vi "define.vi"(8 "error in (no error)":errorcluster, 11 "ColorOverlay in":refnum<class "ColorOverlay.lvclass">) -> (0 "error out":errorcluster, 2 "color cluster out":T2(array[cluster]), 3 "ColorOverlay out":refnum<class "ColorOverlay.lvclass">)   [LabVIEW 2010, in "ColorOverlay.lvclass"]
uses:
  ColorOverlay.lvclass
  <vilib>/Utility/miscctls.llb/LVPointTypeDef.ctl
  ColorOverlay.lvclass/ColorOverlay.ctl
  settings_cluster.ctl
  cursor_cluster.ctl
  enum_color_channel.ctl
panel:
  in  "presets":string(combo)
  in  "range":cluster{dbl, dbl}(slide)={255.0, 255.0} scale=1e-05..0.999999
  out "random image out":T1(plugin-control)
  in  "button: done":bool
  in  "color?":bool=TRUE
  in  "start color":cluster{dbl, dbl, dbl, dbl}(slide)={0.0, 0.0, 255.0, 0.0} scale=1e-10..255.0
  in  "end color":cluster{dbl, dbl, dbl, dbl}(slide)={255.0, 0.0, 0.0, 255.0} scale=1e-10..255.0
  in  "# cold pixels":i32 min=0 max=255
  in  "# hot pixels":i32 min=0 max=255
  in  "color lower limit":u32(colorbox)=16860
  in  "color upper limit":u32(colorbox)=16711680
  out "color bar":u32[](array[colorbox])
  out "graph editor":cluster{"ramp array out":u32[]}[](graph)=[{"ramp array out"=[0, 0, 0, 0, 0, 0, 0, 0, 0, 0, 0, 0, 0, 1, 1, 1, 1, 1, 1, 1, 1, 1, 1, 1, 1, 1, 1, 1, 1, 1, 1, 1, 1, 1, 1, 1, 1, 1, 1, 2, 2, 2, 2, 2, 2, 2, 2, 2, 2, 2, 2, 2, 2, 2, 2, 2, 2, 2, 2, 2, 2, 2, 2, 2, 3, 3, 3, 3, 3, 3, 3, 3, 3, 3, 3, 3, 3, 3, 3, 3, 3, 3, 3, 3, 3, 3, 3, 3, 3, 4, 4, 4, 4, 4, 4, 4, 4, 4, 4, 4, 4, 4, 4, 4, 4, 4, 4, 4, 4, 4, 4, 4, 4, 4, 4, 5, 5, 5, 5, 5, 5, 5, 5, 5, 5, 5, 5, 5, 7, 9, 11, 13, 15, 17, 19, 21, 22, 24, 26, 28, 30, 32, 34, 36, 38, 40, 42, 44, 46, 48, 50, 52, 53, 55, 57, 59, 61, 63, 65, 67, 69, 71, 73, 75, 77, 79, 81, 83, 84, 86, 88, 90, 92, 94, 96, 98, 100, 102, 104, 106, 108, 110, 112, 114, 115, 117, 119, 121, 123, 125, 127, 129, 131, 133, 135, 137, 139, 141, 143, 145, 146, 148, 150, 152, 154, 156, 158, 160, 162, 164, 166, 168, 170, 172, 174, 176, 177, 179, 181, 183, 185, 187, 189, 191, 193, 195, 197, 199, 201, 203, 205, 207, 208, 210, 212, 214, 216, 218, 220, 222, 224, 226, 228, 230, 232, 234, 236, 238, 239, 241, 243, 245, 247, 249, 251, 253]}, {"ramp array out"=[0, 2, 4, 6, 8, 10, 12, 14, 16, 18, 20, 22, 24, 26, 28, 30, 32, 34, 36, 38, 40, 42, 44, 46, 48, 50, 52, 54, 56, 58, 60, 62, 64, 66, 68, 70, 72, 74, 76, 78, 80, 82, 84, 86, 88, 90, 92, 94, 96, 98, 100, 102, 104, 106, 108, 110, 112, 114, 116, 118, 120, 122, 124, 126, 129, 131, 133, 135, 137, 139, 141, 143, 145, 147, 149, 151, 153, 155, 157, 159, 161, 163, 165, 167, 169, 171, 173, 175, 177, 179, 181, 183, 185, 187, 189, 191, 193, 195, 197, 199, 201, 203, 205, 207, 209, 211, 213, 215, 217, 219, 221, 223, 225, 227, 229, 231, 233, 235, 237, 239, 241, 243, 245, 247, 249, 251, 253, 255, 253, 251, 249, 247, 245, 243, 241, 239, 237, 235, 233, 231, 229, 227, 225, 223, 221, 219, 217, 215, 213, 212, 210, 208, 206, 204, 202, 200, 198, 196, 194, 192, 190, 188, 186, 184, 182, 180, 178, 176, 174, 172, 170, 168, 166, 164, 162, 160, 158, 156, 154, 152, 150, 148, 146, 144, 142, 140, 138, 136, 134, 132, 130, 128, 127, 125, 123, 121, 119, 117, 115, 113, 111, 109, 107, 105, 103, 101, 99, 97, 95, 93, 91, 89, 87, 85, 83, 81, 79, 77, 75, 73, 71, 69, 67, 65, 63, 61, 59, 57, 55, 53, 51, 49, 47, 45, 43, 42, 40, 38, 36, 34, 32, 30, 28, 26, 24, 22, 20, 18, 16, 14, 12, 10, 8, 6, 4, 2]}, {"ramp array out"=[255, 253, 251, 249, 247, 245, 243, 241, 239, 237, 235, 233, 231, 229, 227, 225, 224, 222, 220, 218, 216, 214, 212, 210, 208, 206, 204, 202, 200, 198, 196, 194, 192, 190, 188, 186, 184, 182, 180, 178, 176, 174, 172, 170, 168, 166, 164, 162, 161, 159, 157, 155, 153, 151, 149, 147, 145, 143, 141, 139, 137, 135, 133, 131, 129, 127, 125, 123, 121, 119, 117, 115, 113, 111, 109, 107, 105, 103, 101, 99, 98, 96, 94, 92, 90, 88, 86, 84, 82, 80, 78, 76, 74, 72, 70, 68, 66, 64, 62, 60, 58, 56, 54, 52, 50, 48, 46, 44, 42, 40, 38, 36, 35, 33, 31, 29, 27, 25, 23, 21, 19, 17, 15, 13, 11, 9, 7, 5, 5, 5, 5, 5, 5, 5, 5, 5, 5, 5, 5, 5, 4, 4, 4, 4, 4, 4, 4, 4, 4, 4, 4, 4, 4, 4, 4, 4, 4, 4, 4, 4, 4, 4, 4, 4, 4, 4, 3, 3, 3, 3, 3, 3, 3, 3, 3, 3, 3, 3, 3, 3, 3, 3, 3, 3, 3, 3, 3, 3, 3, 3, 3, 3, 2, 2, 2, 2, 2, 2, 2, 2, 2, 2, 2, 2, 2, 2, 2, 2, 2, 2, 2, 2, 2, 2, 2, 2, 2, 2, 1, 1, 1, 1, 1, 1, 1, 1, 1, 1, 1, 1, 1, 1, 1, 1, 1, 1, 1, 1, 1, 1, 1, 1, 1, 1, 0, 0, 0, 0, 0, 0, 0, 0, 0, 0, 0, 0]}, {"ramp array out"=[255, 253, 251, 249, 247, 245, 243, 241, 239, 237, 235, 233, 231, 229, 227, 225, 224, 222, 220, 218, 216, 214, 212, 210, 208, 206, 204, 202, 200, 198, 196, 194, 192, 190, 188, 186, 184, 182, 180, 178, 176, 174, 172, 170, 168, 166, 164, 162, 161, 159, 157, 155, 153, 151, 149, 147, 145, 143, 141, 139, 137, 135, 133, 131, 129, 127, 125, 123, 121, 119, 117, 115, 113, 111, 109, 107, 105, 103, 101, 99, 98, 96, 94, 92, 90, 88, 86, 84, 82, 80, 78, 76, 74, 72, 70, 68, 66, 64, 62, 60, 58, 56, 54, 52, 50, 48, 46, 44, 42, 40, 38, 36, 35, 33, 31, 29, 27, 25, 23, 21, 19, 17, 15, 13, 11, 9, 7, 5, 5, 5, 5, 5, 5, 5, 5, 5, 5, 5, 5, 5, 4, 4, 4, 4, 4, 4, 4, 4, 4, 4, 4, 4, 4, 4, 4, 4, 4, 4, 4, 4, 4, 4, 4, 4, 4, 4, 3, 3, 3, 3, 3, 3, 3, 3, 3, 3, 3, 3, 3, 3, 3, 3, 3, 3, 3, 3, 3, 3, 3, 3, 3, 3, 2, 2, 2, 2, 2, 2, 2, 2, 2, 2, 2, 2, 2, 2, 2, 2, 2, 2, 2, 2, 2, 2, 2, 2, 2, 2, 1, 1, 1, 1, 1, 1, 1, 1, 1, 1, 1, 1, 1, 1, 1, 1, 1, 1, 1, 1, 1, 1, 1, 1, 1, 1, 0, 0, 0, 0, 0, 0, 0, 0, 0, 0, 0, 0]}]
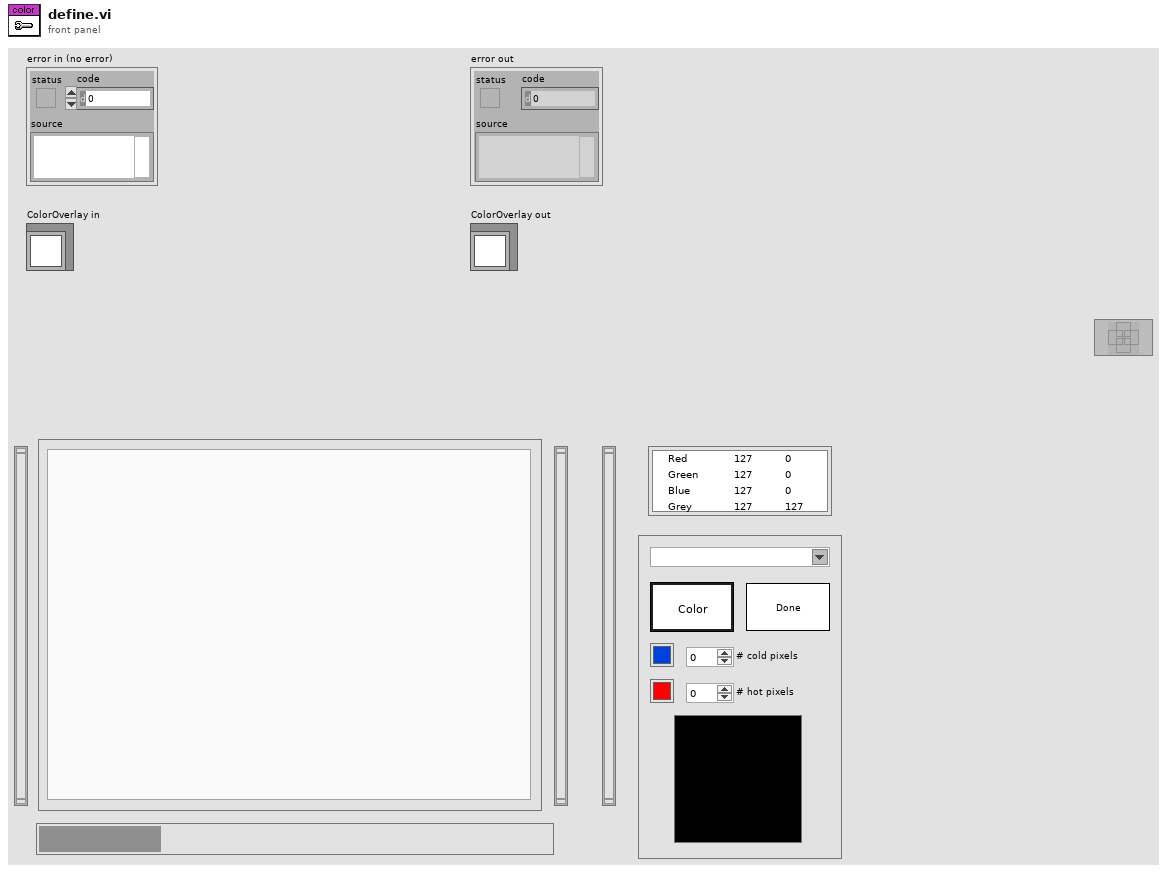
[diagram p1: front panel]
types:
  T1 = typedef "IMAQ Image.ctl" = refnum<image>
  T2 = cluster{"Numeric":u32, "Numeric":u32, "Numeric":u32}[]
  T3 = typedef "LVPointTypeDef.ctl" = cluster{"Horizontal":i16, "Vertical":i16}
  T4 = typedef "ColorOverlay.lvclass/settings_cluster.ctl" = cluster{"# cold pixels":i32, "# hot pixels":i32, "graph editor":cluster{"ramp array out":u32[]}[], "color lower limit":u32, "color upper limit":u32, "color?":bool, "start color":cluster{u8, u8, u8, u8}, "end color":cluster{u8, u8, u8, u8}, "array of cursors":T5[]}
  T5 = typedef "ColorOverlay.lvclass/cursor_cluster.ctl" = cluster{"cursor position":dbl[]}
  T6 = typedef "ColorOverlay.lvclass/enum_color_channel.ctl" = enum16{"red", "green", "blue", "gray"}
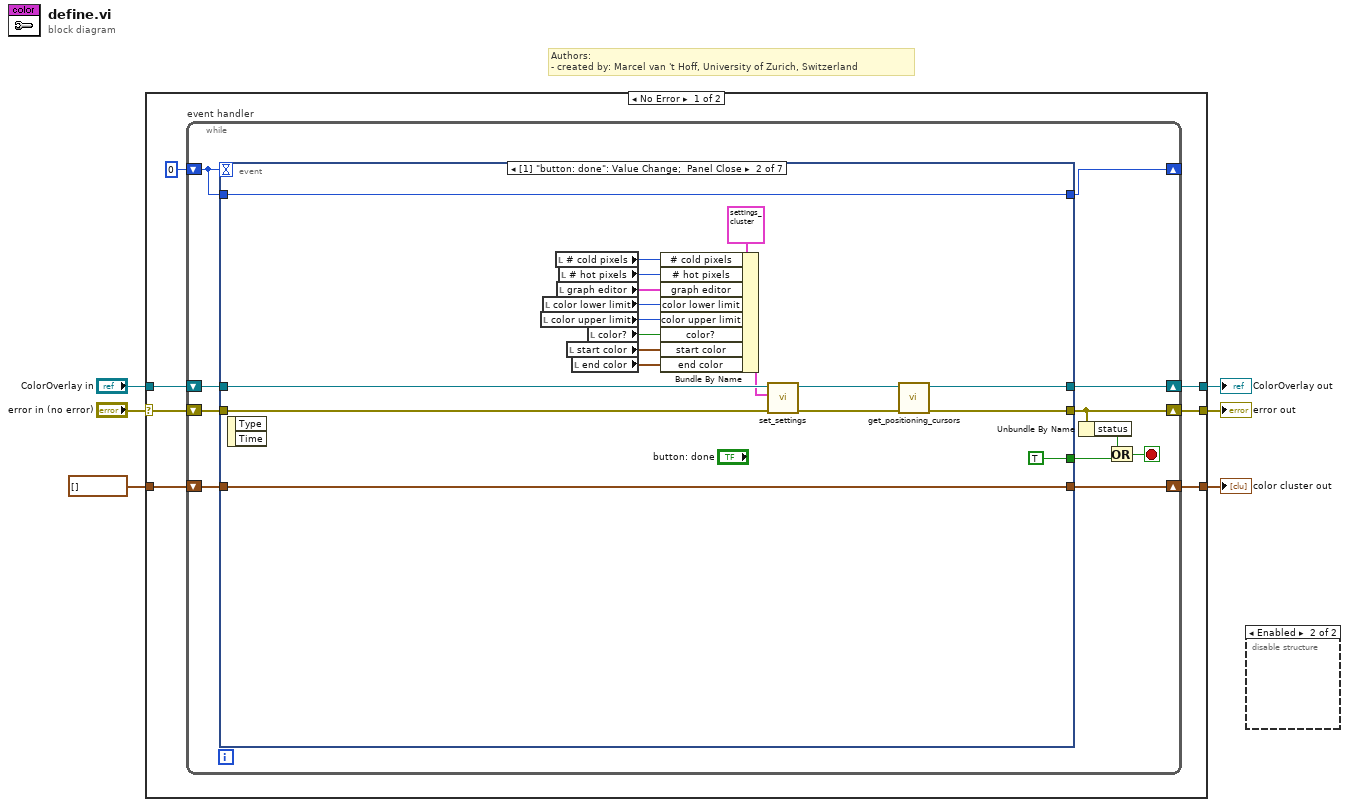
[diagram p0: block diagram]
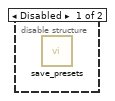
[diagram p2: hidden frame]
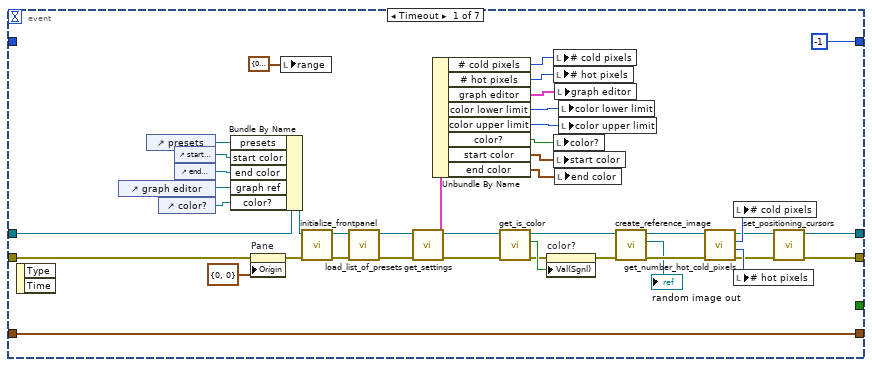
[diagram p3: hidden frame]
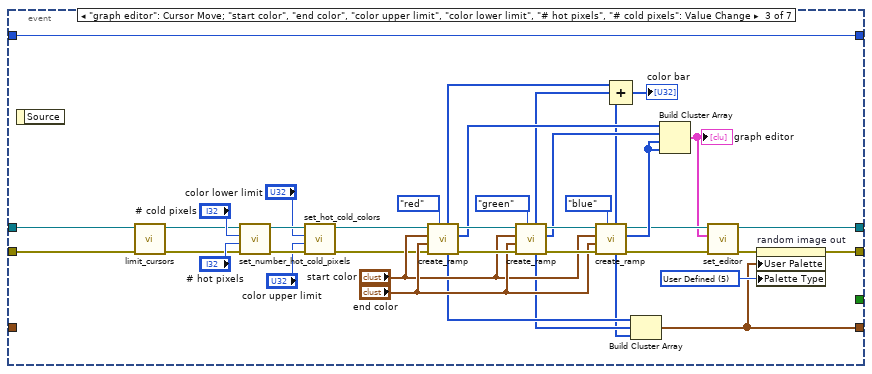
[diagram p4: hidden frame]
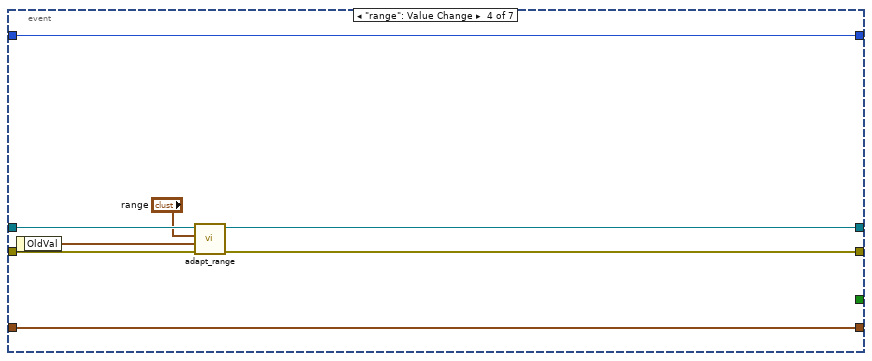
[diagram p5: hidden frame]
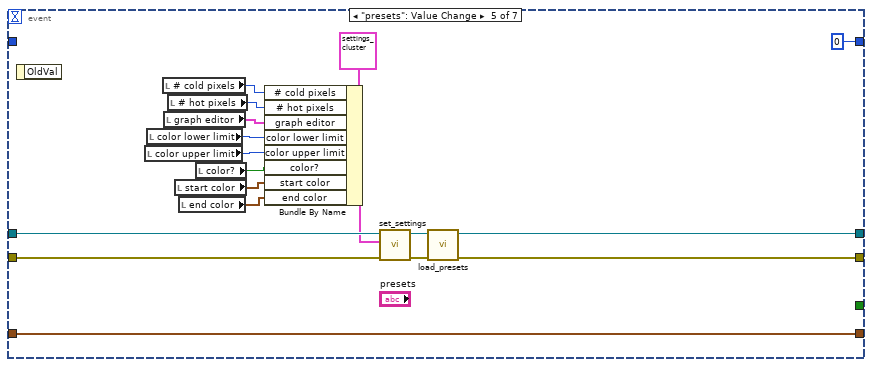
[diagram p6: hidden frame]
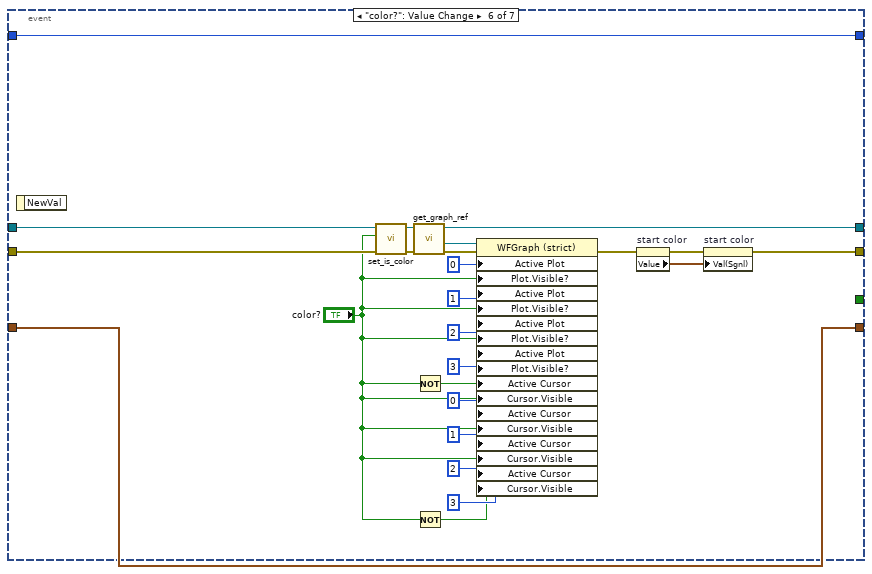
[diagram p7: hidden frame]
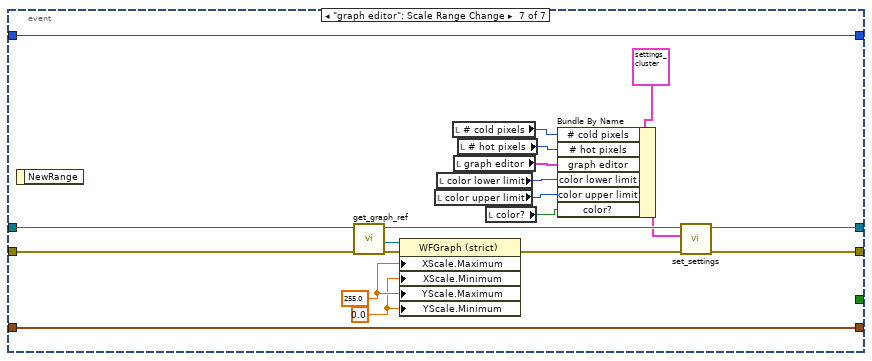
[diagram p8: hidden frame]
diagram:
  # "Authors: \n- created by: Marcel van 't Hoff, University of Zurich, Switzerland"
  n1 = case shown="No Error" "error in (no error)" {
    selector: "error in (no error)" -> [w9 w196]
    tunnel: [w12 w195] -> w4
    tunnel: "ColorOverlay in" -> [w10 w195]
    tunnel: [w13 w196] -> w3
    tunnel: [w8 _] -> w2
    tunnel: T2 [] -> [w7 _]
    frame No Error {
      n2 = while "event handler" {
        shift-right: [w19] -> w13
        shift-left: w9 -> [w24]
        shift-right: [w22] -> w12
        shift-left: w10 -> [w23]
        shift-right: [w20] -> _
        shift-left: 0 -> [w21]
        shift-right: [w14] -> w8
        shift-left: w7 -> [w15]
        stop <- w16 stop-if-true
        n3 = event shown="[1] \"button: done\": Value Change;  Panel Close" {
          selector: _ -> [_ _ _ _ _ _ _]
          dyn-events: _ -> [_ _ _ _ _ _ _]
          timeout: w21 -> [_ _ _ _ _ _ _]
          tunnel: w24 -> [w36 w80 w86 w128 w140 w153 w192]
          tunnel: [w42 w66 w114 w127 w136 w161 w175] -> w19
          tunnel: w23 -> [w62 w81 w88 w130 w141 w155 w191]
          tunnel: [w44 w68 w92 w129 w135 w160 w176] -> w22
          tunnel: w21 -> [_ w84 w115 w132 _ w157 w188]
          tunnel: [-1 w84 w115 w132 0 w157 w188] -> w20
          tunnel: [_ TRUE _ _ _ _ _] -> w17
          tunnel: [w61 w82 w112 w131 w150 w156 w187] -> w14
          tunnel: w15 -> [w61 w82 _ w131 w150 w156 w187]
          event Timeout {
            n4 = event-data() -> ()  [unwired: 1 in, 2 out]
            n5 = control-ref of="graph editor"() -> (w63:refnum<vi>)
            n6 = control-ref of="presets"() -> (w25:refnum<vi>)
            n7 = control-ref of="color?"() -> (w30:refnum<vi>)
            n8 = control-ref of="start color"() -> (w32:refnum<vi>)
            n9 = control-ref of="end color"() -> (w33:refnum<vi>)
            n10 = Bundle By Name(cluster=w62, "presets"=w25, "start color"=w32, "end color"=w33, "graph ref"=w63, "color?"=w30) -> (w64:refnum<class "ColorOverlay.lvclass">)
            n11 = property on="Pane" class="Pane"(error in=w36, "Origin"=T3 {"Horizontal"=0, "Vertical"=0}) -> (error out=w35:errorcluster)  [unwired: 1 in, 1 out]
            n12 = local write "range"(cluster{dbl, dbl} {0.999999, 1e-05} ("range")) -> ()
            n13 = call-dynamic "initialize_frontpanel.vi"("error in (no error)"=w35, "ColorOverlay in"=w64) -> ("error out"=w27:errorcluster, "ColorOverlay out"=w29:refnum<class "ColorOverlay.lvclass">)  [unwired: 8 in]
            n14 = call-dynamic "load_list_of_presets.vi"("error in (no error)"=w27, "ColorOverlay in"=w29) -> ("error out"=w26:errorcluster, "ColorOverlay out"=w28:refnum<class "ColorOverlay.lvclass">)  [unwired: 8 in]
            n15 = call-dynamic "get_settings.vi"("error in (no error)"=w26, "ColorOverlay in"=w28) -> ("error out"=w56:errorcluster, "settings cluster"=w54:T4, "ColorOverlay out"=w55:refnum<class "ColorOverlay.lvclass">)  [unwired: 7 in]
            n16 = Unbundle By Name(w54) -> ("# cold pixels"=w53:i32, "# hot pixels"=w52:i32, "graph editor"=w51:cluster{"ramp array out":u32[]}[], "color lower limit"=w48:u32, "color upper limit"=w49:u32, "color?"=w50:bool, "start color"=w47:cluster{u8, u8, u8, u8}, "end color"=w46:cluster{u8, u8, u8, u8})
            n17 = call-dynamic "get_is_color.vi"("error in (no error)"=w56, "ColorOverlay in"=w55) -> ("error out"=w57:errorcluster, "color?"=w58:bool, "ColorOverlay out"=w41:refnum<class "ColorOverlay.lvclass">)  [unwired: 7 in]
            n18 = property on="color?" class="Bool (strict)"(error in=w57, "Val(Sgnl)"=w58) -> (error out=w39:errorcluster)  [unwired: 1 in, 1 out]
            n19 = local write "# cold pixels"(w53) -> ()
            n20 = local write "# hot pixels"(w52) -> ()
            n21 = local write "color?"(w50) -> ()
            n22 = local write "start color"(w47) -> ()
            n23 = local write "graph editor"(w51) -> ()
            n24 = local write "end color"(w46) -> ()
            n25 = local write "color lower limit"(w48) -> ()
            n26 = local write "color upper limit"(w49) -> ()
            n27 = call-dynamic "create_reference_image.vi"("error in (no error)"=w39, "ColorOverlay in"=w41) -> ("error out"=w38:errorcluster, "reference image out"=→"random image out":T1, "ColorOverlay out"=w40:refnum<class "ColorOverlay.lvclass">)  [unwired: 7 in]
            n28 = call-dynamic "get_number_hot_cold_pixels.vi"("error in (no error)"=w38, "ColorOverlay in"=w40) -> ("error out"=w43:errorcluster, "# hot pixels"=w59:i32, "# cold pixels"=w60:i32, "ColorOverlay out"=w45:refnum<class "ColorOverlay.lvclass">)  [unwired: 6 in]
            n29 = local write "# cold pixels"(w60) -> ()
            n30 = local write "# hot pixels"(w59) -> ()
            n31 = call-dynamic "set_positioning_cursors.vi"("error in (no error)"=w43, "ColorOverlay in"=w45) -> ("error out"=w42:errorcluster, "ColorOverlay out"=w44:refnum<class "ColorOverlay.lvclass">)  [unwired: 8 in]
          }
          event "button: done": Value Change; Panel Close {
            n32 = event-data() -> ()  [unwired: 1 in, 2 out]
            n33 = local read "color upper limit"() -> (w74:u32)
            n34 = local read "color lower limit"() -> (w75:u32)
            n35 = local read "# cold pixels"() -> (w78:i32)
            n36 = local read "graph editor"() -> (w76:cluster{"ramp array out":u32[]}[])
            n37 = local read "# hot pixels"() -> (w77:i32)
            n38 = local read "start color"() -> (w71:cluster{dbl, dbl, dbl, dbl})
            n39 = local read "end color"() -> (w70:cluster{dbl, dbl, dbl, dbl})
            n40 = local read "color?"() -> (w73:bool)
            n41 = Bundle By Name(cluster=T4 {"# cold pixels"=0, "# hot pixels"=0, "graph editor"=[{"ramp array out"=[0, 0, 0, 0, 0, 0, 0, 0, 0, 0, 0, 0, 0, 1, 1, 1, 1, 1, 1, 1, 1, 1, 1, 1, 1, 1, 1, 1, 1, 1, 1, 1, 1, 1, 1, 1, 1, 1, 1, 2, 2, 2, 2, 2, 2, 2, 2, 2, 2, 2, 2, 2, 2, 2, 2, 2, 2, 2, 2, 2, 2, 2, 2, 2, 3, 3, 3, 3, 3, 3, 3, 3, 3, 3, 3, 3, 3, 3, 3, 3, 3, 3, 3, 3, 3, 3, 3, 3, 3, 4, 4, 4, 4, 4, 4, 4, 4, 4, 4, 4, 4, 4, 4, 4, 4, 4, 4, 4, 4, 4, 4, 4, 4, 4, 4, 5, 5, 5, 5, 5, 5, 5, 5, 5, 5, 5, 5, 5, 7, 9, 11, 13, 15, 17, 19, 21, 22, 24, 26, 28, 30, 32, 34, 36, 38, 40, 42, 44, 46, 48, 50, 52, 53, 55, 57, 59, 61, 63, 65, 67, 69, 71, 73, 75, 77, 79, 81, 83, 84, 86, 88, 90, 92, 94, 96, 98, 100, 102, 104, 106, 108, 110, 112, 114, 115, 117, 119, 121, 123, 125, 127, 129, 131, 133, 135, 137, 139, 141, 143, 145, 146, 148, 150, 152, 154, 156, 158, 160, 162, 164, 166, 168, 170, 172, 174, 176, 177, 179, 181, 183, 185, 187, 189, 191, 193, 195, 197, 199, 201, 203, 205, 207, 208, 210, 212, 214, 216, 218, 220, 222, 224, 226, 228, 230, 232, 234, 236, 238, 239, 241, 243, 245, 247, 249, 251, 253]}, {"ramp array out"=[0, 2, 4, 6, 8, 10, 12, 14, 16, 18, 20, 22, 24, 26, 28, 30, 32, 34, 36, 38, 40, 42, 44, 46, 48, 50, 52, 54, 56, 58, 60, 62, 64, 66, 68, 70, 72, 74, 76, 78, 80, 82, 84, 86, 88, 90, 92, 94, 96, 98, 100, 102, 104, 106, 108, 110, 112, 114, 116, 118, 120, 122, 124, 126, 129, 131, 133, 135, 137, 139, 141, 143, 145, 147, 149, 151, 153, 155, 157, 159, 161, 163, 165, 167, 169, 171, 173, 175, 177, 179, 181, 183, 185, 187, 189, 191, 193, 195, 197, 199, 201, 203, 205, 207, 209, 211, 213, 215, 217, 219, 221, 223, 225, 227, 229, 231, 233, 235, 237, 239, 241, 243, 245, 247, 249, 251, 253, 255, 253, 251, 249, 247, 245, 243, 241, 239, 237, 235, 233, 231, 229, 227, 225, 223, 221, 219, 217, 215, 213, 212, 210, 208, 206, 204, 202, 200, 198, 196, 194, 192, 190, 188, 186, 184, 182, 180, 178, 176, 174, 172, 170, 168, 166, 164, 162, 160, 158, 156, 154, 152, 150, 148, 146, 144, 142, 140, 138, 136, 134, 132, 130, 128, 127, 125, 123, 121, 119, 117, 115, 113, 111, 109, 107, 105, 103, 101, 99, 97, 95, 93, 91, 89, 87, 85, 83, 81, 79, 77, 75, 73, 71, 69, 67, 65, 63, 61, 59, 57, 55, 53, 51, 49, 47, 45, 43, 42, 40, 38, 36, 34, 32, 30, 28, 26, 24, 22, 20, 18, 16, 14, 12, 10, 8, 6, 4, 2]}, {"ramp array out"=[255, 253, 251, 249, 247, 245, 243, 241, 239, 237, 235, 233, 231, 229, 227, 225, 224, 222, 220, 218, 216, 214, 212, 210, 208, 206, 204, 202, 200, 198, 196, 194, 192, 190, 188, 186, 184, 182, 180, 178, 176, 174, 172, 170, 168, 166, 164, 162, 161, 159, 157, 155, 153, 151, 149, 147, 145, 143, 141, 139, 137, 135, 133, 131, 129, 127, 125, 123, 121, 119, 117, 115, 113, 111, 109, 107, 105, 103, 101, 99, 98, 96, 94, 92, 90, 88, 86, 84, 82, 80, 78, 76, 74, 72, 70, 68, 66, 64, 62, 60, 58, 56, 54, 52, 50, 48, 46, 44, 42, 40, 38, 36, 35, 33, 31, 29, 27, 25, 23, 21, 19, 17, 15, 13, 11, 9, 7, 5, 5, 5, 5, 5, 5, 5, 5, 5, 5, 5, 5, 5, 4, 4, 4, 4, 4, 4, 4, 4, 4, 4, 4, 4, 4, 4, 4, 4, 4, 4, 4, 4, 4, 4, 4, 4, 4, 4, 3, 3, 3, 3, 3, 3, 3, 3, 3, 3, 3, 3, 3, 3, 3, 3, 3, 3, 3, 3, 3, 3, 3, 3, 3, 3, 2, 2, 2, 2, 2, 2, 2, 2, 2, 2, 2, 2, 2, 2, 2, 2, 2, 2, 2, 2, 2, 2, 2, 2, 2, 2, 1, 1, 1, 1, 1, 1, 1, 1, 1, 1, 1, 1, 1, 1, 1, 1, 1, 1, 1, 1, 1, 1, 1, 1, 1, 1, 0, 0, 0, 0, 0, 0, 0, 0, 0, 0, 0, 0]}, {"ramp array out"=[255, 253, 251, 249, 247, 245, 243, 241, 239, 237, 235, 233, 231, 229, 227, 225, 224, 222, 220, 218, 216, 214, 212, 210, 208, 206, 204, 202, 200, 198, 196, 194, 192, 190, 188, 186, 184, 182, 180, 178, 176, 174, 172, 170, 168, 166, 164, 162, 161, 159, 157, 155, 153, 151, 149, 147, 145, 143, 141, 139, 137, 135, 133, 131, 129, 127, 125, 123, 121, 119, 117, 115, 113, 111, 109, 107, 105, 103, 101, 99, 98, 96, 94, 92, 90, 88, 86, 84, 82, 80, 78, 76, 74, 72, 70, 68, 66, 64, 62, 60, 58, 56, 54, 52, 50, 48, 46, 44, 42, 40, 38, 36, 35, 33, 31, 29, 27, 25, 23, 21, 19, 17, 15, 13, 11, 9, 7, 5, 5, 5, 5, 5, 5, 5, 5, 5, 5, 5, 5, 5, 4, 4, 4, 4, 4, 4, 4, 4, 4, 4, 4, 4, 4, 4, 4, 4, 4, 4, 4, 4, 4, 4, 4, 4, 4, 4, 3, 3, 3, 3, 3, 3, 3, 3, 3, 3, 3, 3, 3, 3, 3, 3, 3, 3, 3, 3, 3, 3, 3, 3, 3, 3, 2, 2, 2, 2, 2, 2, 2, 2, 2, 2, 2, 2, 2, 2, 2, 2, 2, 2, 2, 2, 2, 2, 2, 2, 2, 2, 1, 1, 1, 1, 1, 1, 1, 1, 1, 1, 1, 1, 1, 1, 1, 1, 1, 1, 1, 1, 1, 1, 1, 1, 1, 1, 0, 0, 0, 0, 0, 0, 0, 0, 0, 0, 0, 0]}], "color lower limit"=16860, "color upper limit"=16711680, "color?"=FALSE, "start color"={0, 0, 0, 0}, "end color"={0, 0, 0, 0}, "array of cursors"=[]} ("settings cluster"), "# cold pixels"=w78, "# hot pixels"=w77, "graph editor"=w76, "color lower limit"=w75, "color upper limit"=w74, "color?"=w73, "start color"=w71, "end color"=w70) -> (w72:T4)
            n42 = call-dynamic "set_settings.vi"("error in (no error)"=w80, "settings cluster"=w72, "ColorOverlay in"=w81) -> ("error out"=w67:errorcluster, "ColorOverlay out"=w69:refnum<class "ColorOverlay.lvclass">)  [unwired: 7 in]
            n43 = call-dynamic "get_positioning_cursors.vi"("error in (no error)"=w67, "ColorOverlay in"=w69) -> ("error out"=w66:errorcluster, "ColorOverlay out"=w68:refnum<class "ColorOverlay.lvclass">)  [unwired: 8 in]
          }
          event "graph editor": Cursor Move; "start color", "end color", "color upper limit", "color lower limit", "# hot pixels", "# cold pixels": Value Change {
            w113 = u32 5 items=["Grayscale", "Binary", "Gradient", "Rainbow", "Temperature", "User Defined"] ("Palette:Palette Type")
            n44 = event-data() -> ()  [unwired: 1 in, 1 out]
            n45 = call-dynamic "limit_cursors.vi"("error in (no error)"=w86, "ColorOverlay in"=w88) -> ("error out"=w85:errorcluster, "ColorOverlay out"=w87:refnum<class "ColorOverlay.lvclass">)  [unwired: 8 in]
            n46 = call-dynamic "set_number_hot_cold_pixels.vi"("error in (no error)"=w85, "# hot pixels"="# hot pixels", "# cold pixels"="# cold pixels", "ColorOverlay in"=w87) -> ("error out"=w109:errorcluster, "ColorOverlay out"=w111:refnum<class "ColorOverlay.lvclass">)  [unwired: 6 in]
            n47 = call-dynamic "set_hot_cold_colors.vi"("error in (no error)"=w109, "color higher limit"="color upper limit", "color lower limit"="color lower limit", "ColorOverlay in"=w111) -> ("error out"=w108:errorcluster, "ColorOverlay out"=w110:refnum<class "ColorOverlay.lvclass">)  [unwired: 6 in]
            n48 = call-dynamic "create_ramp.vi"("channel"=enum_color_channel."red", "error in (no error)"=w108, "end color"="end color", "start color"="start color", "ColorOverlay in"=w110) -> ("error out"=w120:errorcluster, "ramp array out"=w107:u32[], "ColorOverlay out"=w119:refnum<class "ColorOverlay.lvclass">, "ramp array out correct dec"=w106:u32[], "ramp array out corrected hex"=w96:u32[])  [unwired: 2 in]
            n49 = call-dynamic "create_ramp.vi"("channel"=enum_color_channel."green", "error in (no error)"=w120, "end color"="end color", "start color"="start color", "ColorOverlay in"=w119) -> ("error out"=w121:errorcluster, "ramp array out"=w103:u32[], "ColorOverlay out"=w118:refnum<class "ColorOverlay.lvclass">, "ramp array out correct dec"=w105:u32[], "ramp array out corrected hex"=w95:u32[])  [unwired: 2 in]
            n50 = call-dynamic "create_ramp.vi"("channel"=enum_color_channel."blue", "error in (no error)"=w121, "end color"="end color", "start color"="start color", "ColorOverlay in"=w118) -> ("error out"=w90:errorcluster, "ramp array out"=w102:u32[], "ColorOverlay out"=w93:refnum<class "ColorOverlay.lvclass">, "ramp array out correct dec"=w104:u32[], "ramp array out corrected hex"=w94:u32[])  [unwired: 2 in]
            n51 = Compound Arithmetic op=ADD(w96, w95, w94) -> (→"color bar":u32[])
            n52 = Build Cluster Array(w106, w105, w104) -> (w112:T2)
            n53 = Build Cluster Array(w107, w103, w102, w102) -> (w91:cluster{"ramp array out":u32[]}[])
            "graph editor" <- w91
            n54 = call-dynamic "set_editor.vi"("error in (no error)"=w90, "graph editor"=w91, "ColorOverlay in"=w93) -> ("error out"=w89:errorcluster, "ColorOverlay out"=w92:refnum<class "ColorOverlay.lvclass">)  [unwired: 7 in]
            n55 = property on="random image out" class="ImageControl"(error in=w89, "User Palette"=w112, "Palette Type"=w113) -> (error out=w114:errorcluster)  [unwired: 1 in, 1 out]
          }
          event "range": Value Change {
            n56 = event-data() -> ("OldVal"=w126:cluster{dbl, dbl})  [unwired: 1 in]
            n57 = call-dynamic "adapt_range.vi"("error in (no error)"=w128, "range old"=w126, "range new"="range", "ColorOverlay in"=w130) -> ("error out"=w127:errorcluster, "ColorOverlay out"=w129:refnum<class "ColorOverlay.lvclass">)  [unwired: 6 in]
          }
          event "presets": Value Change {
            n58 = event-data() -> ()  [unwired: 1 in, 1 out]
            n59 = local read "color upper limit"() -> (w146:u32)
            n60 = local read "color lower limit"() -> (w147:u32)
            n61 = local read "# cold pixels"() -> (w149:i32)
            n62 = local read "graph editor"() -> (w138:cluster{"ramp array out":u32[]}[])
            n63 = local read "# hot pixels"() -> (w148:i32)
            n64 = local read "start color"() -> (w144:cluster{dbl, dbl, dbl, dbl})
            n65 = local read "end color"() -> (w143:cluster{dbl, dbl, dbl, dbl})
            n66 = local read "color?"() -> (w145:bool)
            n67 = Bundle By Name(cluster=T4 {"# cold pixels"=0, "# hot pixels"=0, "graph editor"=[{"ramp array out"=[0, 0, 0, 0, 0, 0, 0, 0, 0, 0, 0, 0, 0, 1, 1, 1, 1, 1, 1, 1, 1, 1, 1, 1, 1, 1, 1, 1, 1, 1, 1, 1, 1, 1, 1, 1, 1, 1, 1, 2, 2, 2, 2, 2, 2, 2, 2, 2, 2, 2, 2, 2, 2, 2, 2, 2, 2, 2, 2, 2, 2, 2, 2, 2, 3, 3, 3, 3, 3, 3, 3, 3, 3, 3, 3, 3, 3, 3, 3, 3, 3, 3, 3, 3, 3, 3, 3, 3, 3, 4, 4, 4, 4, 4, 4, 4, 4, 4, 4, 4, 4, 4, 4, 4, 4, 4, 4, 4, 4, 4, 4, 4, 4, 4, 4, 5, 5, 5, 5, 5, 5, 5, 5, 5, 5, 5, 5, 5, 7, 9, 11, 13, 15, 17, 19, 21, 22, 24, 26, 28, 30, 32, 34, 36, 38, 40, 42, 44, 46, 48, 50, 52, 53, 55, 57, 59, 61, 63, 65, 67, 69, 71, 73, 75, 77, 79, 81, 83, 84, 86, 88, 90, 92, 94, 96, 98, 100, 102, 104, 106, 108, 110, 112, 114, 115, 117, 119, 121, 123, 125, 127, 129, 131, 133, 135, 137, 139, 141, 143, 145, 146, 148, 150, 152, 154, 156, 158, 160, 162, 164, 166, 168, 170, 172, 174, 176, 177, 179, 181, 183, 185, 187, 189, 191, 193, 195, 197, 199, 201, 203, 205, 207, 208, 210, 212, 214, 216, 218, 220, 222, 224, 226, 228, 230, 232, 234, 236, 238, 239, 241, 243, 245, 247, 249, 251, 253]}, {"ramp array out"=[0, 2, 4, 6, 8, 10, 12, 14, 16, 18, 20, 22, 24, 26, 28, 30, 32, 34, 36, 38, 40, 42, 44, 46, 48, 50, 52, 54, 56, 58, 60, 62, 64, 66, 68, 70, 72, 74, 76, 78, 80, 82, 84, 86, 88, 90, 92, 94, 96, 98, 100, 102, 104, 106, 108, 110, 112, 114, 116, 118, 120, 122, 124, 126, 129, 131, 133, 135, 137, 139, 141, 143, 145, 147, 149, 151, 153, 155, 157, 159, 161, 163, 165, 167, 169, 171, 173, 175, 177, 179, 181, 183, 185, 187, 189, 191, 193, 195, 197, 199, 201, 203, 205, 207, 209, 211, 213, 215, 217, 219, 221, 223, 225, 227, 229, 231, 233, 235, 237, 239, 241, 243, 245, 247, 249, 251, 253, 255, 253, 251, 249, 247, 245, 243, 241, 239, 237, 235, 233, 231, 229, 227, 225, 223, 221, 219, 217, 215, 213, 212, 210, 208, 206, 204, 202, 200, 198, 196, 194, 192, 190, 188, 186, 184, 182, 180, 178, 176, 174, 172, 170, 168, 166, 164, 162, 160, 158, 156, 154, 152, 150, 148, 146, 144, 142, 140, 138, 136, 134, 132, 130, 128, 127, 125, 123, 121, 119, 117, 115, 113, 111, 109, 107, 105, 103, 101, 99, 97, 95, 93, 91, 89, 87, 85, 83, 81, 79, 77, 75, 73, 71, 69, 67, 65, 63, 61, 59, 57, 55, 53, 51, 49, 47, 45, 43, 42, 40, 38, 36, 34, 32, 30, 28, 26, 24, 22, 20, 18, 16, 14, 12, 10, 8, 6, 4, 2]}, {"ramp array out"=[255, 253, 251, 249, 247, 245, 243, 241, 239, 237, 235, 233, 231, 229, 227, 225, 224, 222, 220, 218, 216, 214, 212, 210, 208, 206, 204, 202, 200, 198, 196, 194, 192, 190, 188, 186, 184, 182, 180, 178, 176, 174, 172, 170, 168, 166, 164, 162, 161, 159, 157, 155, 153, 151, 149, 147, 145, 143, 141, 139, 137, 135, 133, 131, 129, 127, 125, 123, 121, 119, 117, 115, 113, 111, 109, 107, 105, 103, 101, 99, 98, 96, 94, 92, 90, 88, 86, 84, 82, 80, 78, 76, 74, 72, 70, 68, 66, 64, 62, 60, 58, 56, 54, 52, 50, 48, 46, 44, 42, 40, 38, 36, 35, 33, 31, 29, 27, 25, 23, 21, 19, 17, 15, 13, 11, 9, 7, 5, 5, 5, 5, 5, 5, 5, 5, 5, 5, 5, 5, 5, 4, 4, 4, 4, 4, 4, 4, 4, 4, 4, 4, 4, 4, 4, 4, 4, 4, 4, 4, 4, 4, 4, 4, 4, 4, 4, 3, 3, 3, 3, 3, 3, 3, 3, 3, 3, 3, 3, 3, 3, 3, 3, 3, 3, 3, 3, 3, 3, 3, 3, 3, 3, 2, 2, 2, 2, 2, 2, 2, 2, 2, 2, 2, 2, 2, 2, 2, 2, 2, 2, 2, 2, 2, 2, 2, 2, 2, 2, 1, 1, 1, 1, 1, 1, 1, 1, 1, 1, 1, 1, 1, 1, 1, 1, 1, 1, 1, 1, 1, 1, 1, 1, 1, 1, 0, 0, 0, 0, 0, 0, 0, 0, 0, 0, 0, 0]}, {"ramp array out"=[255, 253, 251, 249, 247, 245, 243, 241, 239, 237, 235, 233, 231, 229, 227, 225, 224, 222, 220, 218, 216, 214, 212, 210, 208, 206, 204, 202, 200, 198, 196, 194, 192, 190, 188, 186, 184, 182, 180, 178, 176, 174, 172, 170, 168, 166, 164, 162, 161, 159, 157, 155, 153, 151, 149, 147, 145, 143, 141, 139, 137, 135, 133, 131, 129, 127, 125, 123, 121, 119, 117, 115, 113, 111, 109, 107, 105, 103, 101, 99, 98, 96, 94, 92, 90, 88, 86, 84, 82, 80, 78, 76, 74, 72, 70, 68, 66, 64, 62, 60, 58, 56, 54, 52, 50, 48, 46, 44, 42, 40, 38, 36, 35, 33, 31, 29, 27, 25, 23, 21, 19, 17, 15, 13, 11, 9, 7, 5, 5, 5, 5, 5, 5, 5, 5, 5, 5, 5, 5, 5, 4, 4, 4, 4, 4, 4, 4, 4, 4, 4, 4, 4, 4, 4, 4, 4, 4, 4, 4, 4, 4, 4, 4, 4, 4, 4, 3, 3, 3, 3, 3, 3, 3, 3, 3, 3, 3, 3, 3, 3, 3, 3, 3, 3, 3, 3, 3, 3, 3, 3, 3, 3, 2, 2, 2, 2, 2, 2, 2, 2, 2, 2, 2, 2, 2, 2, 2, 2, 2, 2, 2, 2, 2, 2, 2, 2, 2, 2, 1, 1, 1, 1, 1, 1, 1, 1, 1, 1, 1, 1, 1, 1, 1, 1, 1, 1, 1, 1, 1, 1, 1, 1, 1, 1, 0, 0, 0, 0, 0, 0, 0, 0, 0, 0, 0, 0]}], "color lower limit"=16860, "color upper limit"=16711680, "color?"=FALSE, "start color"={0, 0, 0, 0}, "end color"={0, 0, 0, 0}, "array of cursors"=[]} ("settings cluster"), "# cold pixels"=w149, "# hot pixels"=w148, "graph editor"=w138, "color lower limit"=w147, "color upper limit"=w146, "color?"=w145, "start color"=w144, "end color"=w143) -> (w139:T4)
            n68 = call-dynamic "set_settings.vi"("error in (no error)"=w140, "settings cluster"=w139, "ColorOverlay in"=w141) -> ("error out"=w134:errorcluster, "ColorOverlay out"=w133:refnum<class "ColorOverlay.lvclass">)  [unwired: 7 in]
            n69 = call-dynamic "load_presets.vi"("error in (no error)"=w134, "ColorOverlay in"=w133) -> ("error out"=w136:errorcluster, "ColorOverlay out"=w135:refnum<class "ColorOverlay.lvclass">)  [unwired: 8 in]
          }
          event "color?": Value Change {
            n70 = event-data() -> ()  [unwired: 1 in, 1 out]
            n71 = call-dynamic "set_is_color.vi"("error in (no error)"=w153, "color?"="color?", "ColorOverlay in"=w155) -> ("error out"=w152:errorcluster, "ColorOverlay out"=w154:refnum<class "ColorOverlay.lvclass">)  [unwired: 7 in]
            n72 = call-dynamic "get_graph_ref.vi"("error in (no error)"=w152, "ColorOverlay in"=w154) -> ("error out"=w159:errorcluster, "graph ref"=w158:refnum<vi>, "ColorOverlay out"=w160:refnum<class "ColorOverlay.lvclass">)  [unwired: 7 in]
            n73 = Not(x="color?") -> (.not. x?=w170:bool)
            n74 = Not(x="color?") -> (.not. x?=w165:bool)
            n75 = property class="WFGraph (strict)"(reference=w158, error in=w159, "Active Plot"=u32 0, "Plot.Visible?"="color?", "Active Plot"=u32 1, "Plot.Visible?"="color?", "Active Plot"=u32 2, "Plot.Visible?"="color?", "Active Plot"=u32 3, "Plot.Visible?"=w170, "Active Cursor"=u32 0, "Cursor.Visible"="color?", "Active Cursor"=u32 1, "Cursor.Visible"="color?", "Active Cursor"=u32 2, "Cursor.Visible"="color?", "Active Cursor"=u32 3, "Cursor.Visible"=w165) -> (error out=w162:errorcluster)  [unwired: 1 out]
            n76 = property on="start color" class="Slide (strict)"(error in=w162) -> (error out=w164:errorcluster, "Value"=w163:cluster{dbl, dbl, dbl, dbl})  [unwired: 1 in, 1 out]
            n77 = property on="start color" class="Slide (strict)"(error in=w164, "Val(Sgnl)"=w163) -> (error out=w161:errorcluster)  [unwired: 1 in, 1 out]
          }
          event "graph editor": Scale Range Change {
            w189 = 0.0 ("X Scale.Range:Maximum")
            w190 = 255.0 ("X Scale.Range:Maximum")
            n78 = event-data() -> ()  [unwired: 1 in, 1 out]
            n79 = call-dynamic "get_graph_ref.vi"("error in (no error)"=w192, "ColorOverlay in"=w191) -> ("error out"=w193:errorcluster, "graph ref"=w194:refnum<vi>, "ColorOverlay out"=w186:refnum<class "ColorOverlay.lvclass">)  [unwired: 7 in]
            n80 = property class="WFGraph (strict)"(reference=w194, error in=w193, "XScale.Maximum"=w190, "XScale.Minimum"=w189, "YScale.Maximum"=w190, "YScale.Minimum"=w189) -> (error out=w185:errorcluster)  [unwired: 1 out]
            n81 = local read "color upper limit"() -> (w181:u32)
            n82 = local read "color lower limit"() -> (w180:u32)
            n83 = local read "# cold pixels"() -> (w183:i32)
            n84 = local read "graph editor"() -> (w179:cluster{"ramp array out":u32[]}[])
            n85 = local read "# hot pixels"() -> (w178:i32)
            n86 = local read "color?"() -> (w182:bool)
            n87 = Bundle By Name(cluster=T4 {"# cold pixels"=0, "# hot pixels"=0, "graph editor"=[{"ramp array out"=[0, 0, 0, 0, 0, 0, 0, 0, 0, 0, 0, 0, 0, 1, 1, 1, 1, 1, 1, 1, 1, 1, 1, 1, 1, 1, 1, 1, 1, 1, 1, 1, 1, 1, 1, 1, 1, 1, 1, 2, 2, 2, 2, 2, 2, 2, 2, 2, 2, 2, 2, 2, 2, 2, 2, 2, 2, 2, 2, 2, 2, 2, 2, 2, 3, 3, 3, 3, 3, 3, 3, 3, 3, 3, 3, 3, 3, 3, 3, 3, 3, 3, 3, 3, 3, 3, 3, 3, 3, 4, 4, 4, 4, 4, 4, 4, 4, 4, 4, 4, 4, 4, 4, 4, 4, 4, 4, 4, 4, 4, 4, 4, 4, 4, 4, 5, 5, 5, 5, 5, 5, 5, 5, 5, 5, 5, 5, 5, 7, 9, 11, 13, 15, 17, 19, 21, 22, 24, 26, 28, 30, 32, 34, 36, 38, 40, 42, 44, 46, 48, 50, 52, 53, 55, 57, 59, 61, 63, 65, 67, 69, 71, 73, 75, 77, 79, 81, 83, 84, 86, 88, 90, 92, 94, 96, 98, 100, 102, 104, 106, 108, 110, 112, 114, 115, 117, 119, 121, 123, 125, 127, 129, 131, 133, 135, 137, 139, 141, 143, 145, 146, 148, 150, 152, 154, 156, 158, 160, 162, 164, 166, 168, 170, 172, 174, 176, 177, 179, 181, 183, 185, 187, 189, 191, 193, 195, 197, 199, 201, 203, 205, 207, 208, 210, 212, 214, 216, 218, 220, 222, 224, 226, 228, 230, 232, 234, 236, 238, 239, 241, 243, 245, 247, 249, 251, 253]}, {"ramp array out"=[0, 2, 4, 6, 8, 10, 12, 14, 16, 18, 20, 22, 24, 26, 28, 30, 32, 34, 36, 38, 40, 42, 44, 46, 48, 50, 52, 54, 56, 58, 60, 62, 64, 66, 68, 70, 72, 74, 76, 78, 80, 82, 84, 86, 88, 90, 92, 94, 96, 98, 100, 102, 104, 106, 108, 110, 112, 114, 116, 118, 120, 122, 124, 126, 129, 131, 133, 135, 137, 139, 141, 143, 145, 147, 149, 151, 153, 155, 157, 159, 161, 163, 165, 167, 169, 171, 173, 175, 177, 179, 181, 183, 185, 187, 189, 191, 193, 195, 197, 199, 201, 203, 205, 207, 209, 211, 213, 215, 217, 219, 221, 223, 225, 227, 229, 231, 233, 235, 237, 239, 241, 243, 245, 247, 249, 251, 253, 255, 253, 251, 249, 247, 245, 243, 241, 239, 237, 235, 233, 231, 229, 227, 225, 223, 221, 219, 217, 215, 213, 212, 210, 208, 206, 204, 202, 200, 198, 196, 194, 192, 190, 188, 186, 184, 182, 180, 178, 176, 174, 172, 170, 168, 166, 164, 162, 160, 158, 156, 154, 152, 150, 148, 146, 144, 142, 140, 138, 136, 134, 132, 130, 128, 127, 125, 123, 121, 119, 117, 115, 113, 111, 109, 107, 105, 103, 101, 99, 97, 95, 93, 91, 89, 87, 85, 83, 81, 79, 77, 75, 73, 71, 69, 67, 65, 63, 61, 59, 57, 55, 53, 51, 49, 47, 45, 43, 42, 40, 38, 36, 34, 32, 30, 28, 26, 24, 22, 20, 18, 16, 14, 12, 10, 8, 6, 4, 2]}, {"ramp array out"=[255, 253, 251, 249, 247, 245, 243, 241, 239, 237, 235, 233, 231, 229, 227, 225, 224, 222, 220, 218, 216, 214, 212, 210, 208, 206, 204, 202, 200, 198, 196, 194, 192, 190, 188, 186, 184, 182, 180, 178, 176, 174, 172, 170, 168, 166, 164, 162, 161, 159, 157, 155, 153, 151, 149, 147, 145, 143, 141, 139, 137, 135, 133, 131, 129, 127, 125, 123, 121, 119, 117, 115, 113, 111, 109, 107, 105, 103, 101, 99, 98, 96, 94, 92, 90, 88, 86, 84, 82, 80, 78, 76, 74, 72, 70, 68, 66, 64, 62, 60, 58, 56, 54, 52, 50, 48, 46, 44, 42, 40, 38, 36, 35, 33, 31, 29, 27, 25, 23, 21, 19, 17, 15, 13, 11, 9, 7, 5, 5, 5, 5, 5, 5, 5, 5, 5, 5, 5, 5, 5, 4, 4, 4, 4, 4, 4, 4, 4, 4, 4, 4, 4, 4, 4, 4, 4, 4, 4, 4, 4, 4, 4, 4, 4, 4, 4, 3, 3, 3, 3, 3, 3, 3, 3, 3, 3, 3, 3, 3, 3, 3, 3, 3, 3, 3, 3, 3, 3, 3, 3, 3, 3, 2, 2, 2, 2, 2, 2, 2, 2, 2, 2, 2, 2, 2, 2, 2, 2, 2, 2, 2, 2, 2, 2, 2, 2, 2, 2, 1, 1, 1, 1, 1, 1, 1, 1, 1, 1, 1, 1, 1, 1, 1, 1, 1, 1, 1, 1, 1, 1, 1, 1, 1, 1, 0, 0, 0, 0, 0, 0, 0, 0, 0, 0, 0, 0]}, {"ramp array out"=[255, 253, 251, 249, 247, 245, 243, 241, 239, 237, 235, 233, 231, 229, 227, 225, 224, 222, 220, 218, 216, 214, 212, 210, 208, 206, 204, 202, 200, 198, 196, 194, 192, 190, 188, 186, 184, 182, 180, 178, 176, 174, 172, 170, 168, 166, 164, 162, 161, 159, 157, 155, 153, 151, 149, 147, 145, 143, 141, 139, 137, 135, 133, 131, 129, 127, 125, 123, 121, 119, 117, 115, 113, 111, 109, 107, 105, 103, 101, 99, 98, 96, 94, 92, 90, 88, 86, 84, 82, 80, 78, 76, 74, 72, 70, 68, 66, 64, 62, 60, 58, 56, 54, 52, 50, 48, 46, 44, 42, 40, 38, 36, 35, 33, 31, 29, 27, 25, 23, 21, 19, 17, 15, 13, 11, 9, 7, 5, 5, 5, 5, 5, 5, 5, 5, 5, 5, 5, 5, 5, 4, 4, 4, 4, 4, 4, 4, 4, 4, 4, 4, 4, 4, 4, 4, 4, 4, 4, 4, 4, 4, 4, 4, 4, 4, 4, 3, 3, 3, 3, 3, 3, 3, 3, 3, 3, 3, 3, 3, 3, 3, 3, 3, 3, 3, 3, 3, 3, 3, 3, 3, 3, 2, 2, 2, 2, 2, 2, 2, 2, 2, 2, 2, 2, 2, 2, 2, 2, 2, 2, 2, 2, 2, 2, 2, 2, 2, 2, 1, 1, 1, 1, 1, 1, 1, 1, 1, 1, 1, 1, 1, 1, 1, 1, 1, 1, 1, 1, 1, 1, 1, 1, 1, 1, 0, 0, 0, 0, 0, 0, 0, 0, 0, 0, 0, 0]}], "color lower limit"=16860, "color upper limit"=16711680, "color?"=FALSE, "start color"={0, 0, 0, 0}, "end color"={0, 0, 0, 0}, "array of cursors"=[]} ("settings cluster"), "# cold pixels"=w183, "# hot pixels"=w178, "graph editor"=w179, "color lower limit"=w180, "color upper limit"=w181, "color?"=w182) -> (w177:T4)
            n88 = call-dynamic "set_settings.vi"("error in (no error)"=w185, "settings cluster"=w177, "ColorOverlay in"=w186) -> ("error out"=w175:errorcluster, "ColorOverlay out"=w176:refnum<class "ColorOverlay.lvclass">)  [unwired: 7 in]
          }
        }
        n89 = Unbundle By Name(w19) -> ("status"=w18:bool)
        n90 = Or(x=w18, y=w17) -> (x .or. y?=w16:bool)
      }
    }
    frame Error {
    }
  }
  "error out" <- w3
  "ColorOverlay out" <- w4
  "color cluster out" <- w2
  n91 = disable-structure shown="Enabled" {
    frame Disabled {
      n92 = call-dynamic "save_presets.vi"() -> ()  [unwired: 10 in, 2 out]
    }
    frame Enabled {
    }
  }
